vi "Pose3d_New_Default.vi"() -> (3 "outPose3d":T1={"Translation3d"={"X"=0.0, "Y"=0.0, "Z"=0.0}, "Rotation3d"={"Q_quaternion"={"R"=1.0, "V"=[0.0, 0.0, 0.0]}}} {"Translation3d"."Z" format="%14.3f"; "Translation3d"."Y" format="%14.3f"; "Translation3d"."X" format="%14.3f"})   [LabVIEW 2019, in "Trajectory_Library.lvlib"]
doc: "Constructs a pose at the origin facing toward the positive X axis.\n\nParameters:\n -- none --\n\nReturn:\n - POSE3d - Pose3d data structure"
uses:
  Trajectory_Library.lvlib
  TypeDef/TRANSLATION3D.ctl
  TypeDef/QUATERNION.ctl
  TypeDef/ROTATION3D.ctl
  TypeDef/POSE3D.ctl
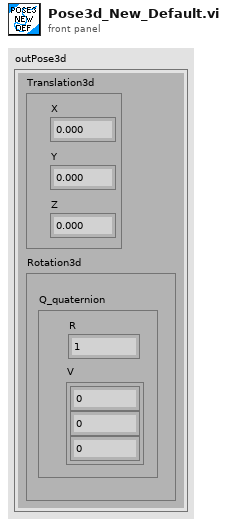
[diagram p1: front panel]
types:
  T1 = typedef "Trajectory_Library.lvlib/POSE3D.ctl" = cluster{"Translation3d":T2, "Rotation3d":T3}
  T2 = typedef "Trajectory_Library.lvlib/TRANSLATION3D.ctl" = cluster{"X":dbl, "Y":dbl, "Z":dbl}
  T3 = typedef "Trajectory_Library.lvlib/ROTATION3D.ctl" = cluster{"Q_quaternion":T4}
  T4 = typedef "Trajectory_Library.lvlib/QUATERNION.ctl" = cluster{"R":dbl, "V":dbl[]}
  T5 = typedef "WPILib_Math.lvlib/TRANSLATION3D.ctl" = cluster{"X":dbl, "Y":dbl, "Z":dbl}
  T6 = typedef "WPILib_Math.lvlib/ROTATION3D.ctl" = cluster{"Q_quaternion":T7}
  T7 = typedef "WPILib_Math.lvlib/QUATERNION.ctl" = cluster{"R":dbl, "V":dbl[]}
  T8 = typedef "WPILib_Math.lvlib/POSE3D.ctl" = cluster{"Translation3d":T5, "Rotation3d":T6}
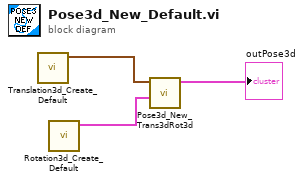
[diagram p0: block diagram]
diagram:
  n1 = call "Translation3d_Create_Default.vi"() -> ("TRANSLATION3D"=w3:T5)  [unwired: 11 in]
  n2 = call "Rotation3d_Create_Default.vi"() -> ("ROTATION3D"=w2:T6)  [unwired: 11 in]
  n3 = call "Pose3d_New_Trans3dRot3d.vi"("Rotation3d"=w2, "Translation3d"=w3) -> ("outPose3d"=→"outPose3d":T8)  [unwired: 9 in]
